vi "_CSM - Read Log Filter Rules - v1.0.vi"(5 "Section Name(\"LogFilterRules\")":string="LogFilterRules", 7 "error in (no error)":errorcluster) -> (1 "error out":errorcluster, 3 "Rules-v1":T1)   [LabVIEW 2017, in "INI-Static-Variable-Support.lvlib"]
uses:
  INI-Static-Variable-Support.lvlib
  <userlib>/_NEVSTOP/Communicable State Machine(CSM)/_Support/Typedef/_CSM_GlobalLog Filter Rules - v1.0.ctl
  <userlib>/_NEVSTOP/Communicable State Machine(CSM)/_Support/Typedef/_CSM_GlobalLog_MSG_TYPE.ctl
  <userlib>/_NEVSTOP/Communicable State Machine(CSM)/_Support/Typedef/_CSM_GlobalLog_STATE_TYPE.ctl
  _fgv-oper.ctl
  <userlib>/_NEVSTOP/Communicable State Machine(CSM)/_Support/ChangeFlag/ChangeFlag-Read.vi
  <userlib>/_NEVSTOP/Communicable State Machine(CSM)/_Support/ChangeFlag/ChangeFlagDB.vi
  <userlib>/_NEVSTOP/Communicable State Machine(CSM)/Communicable State Machine.lvlib
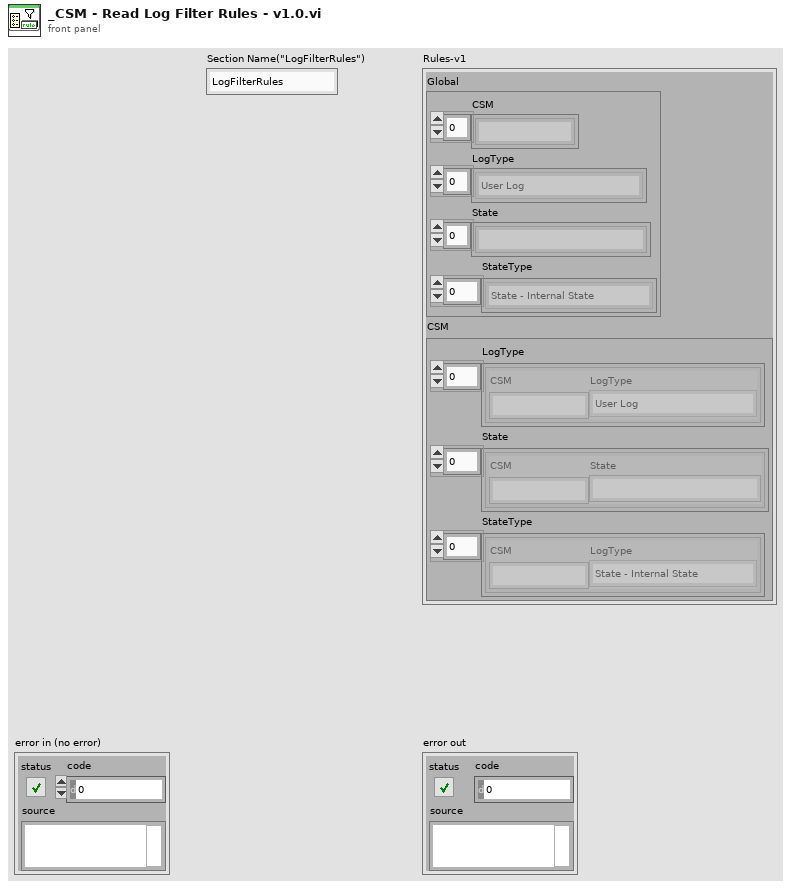
[diagram p1: front panel]
types:
  T1 = typedef "Communicable State Machine.lvlib/_CSM_GlobalLog Filter Rules - v1.0.ctl" = cluster{"Global":cluster{"CSM":string[], "LogType":T2[], "State":string[], "StateType":T3[]}, "CSM":cluster{"LogType":cluster{"CSM":string, "LogType":T2}[], "State":cluster{"CSM":string, "State":string}[], "StateType":cluster{"CSM":string, "LogType":T3}[]}}
  T2 = typedef "Communicable State Machine.lvlib/_CSM_GlobalLog_MSG_TYPE.ctl" = enum16{"User Log", "State Change", "Status", "Interrupt", "Register", "Unregister", "Error Log", "Module Created", "Module Destroyed"}
  T3 = typedef "Communicable State Machine.lvlib/_CSM_GlobalLog_STATE_TYPE.ctl" = enum16{"State - Internal State", "State - External Message", "State - Response", "State - Complete"}
  T4 = typedef "INI-Static-Variable-Support.lvlib/_fgv-oper.ctl" = enum16{"Read", "Write", "Sync", "Sessions", "List Keys", "Load", "List Files", "List Variables", "List Permanent Variables", "Mark Temp Variable as Permenent", "unload", "INIConfig(Memory)", "Reset", "Restore Variable Value"}
  T5 = typedef "LabVIEW-Config.lvlib/Config.ctl" = cluster{"Path":path, "Lines":string[], "Tokens":T6[], "Modified?":bool}
  T6 = typedef "LabVIEW-Config.lvlib/LineToken.ctl" = enum8{"comment", "section", "key", "more"}
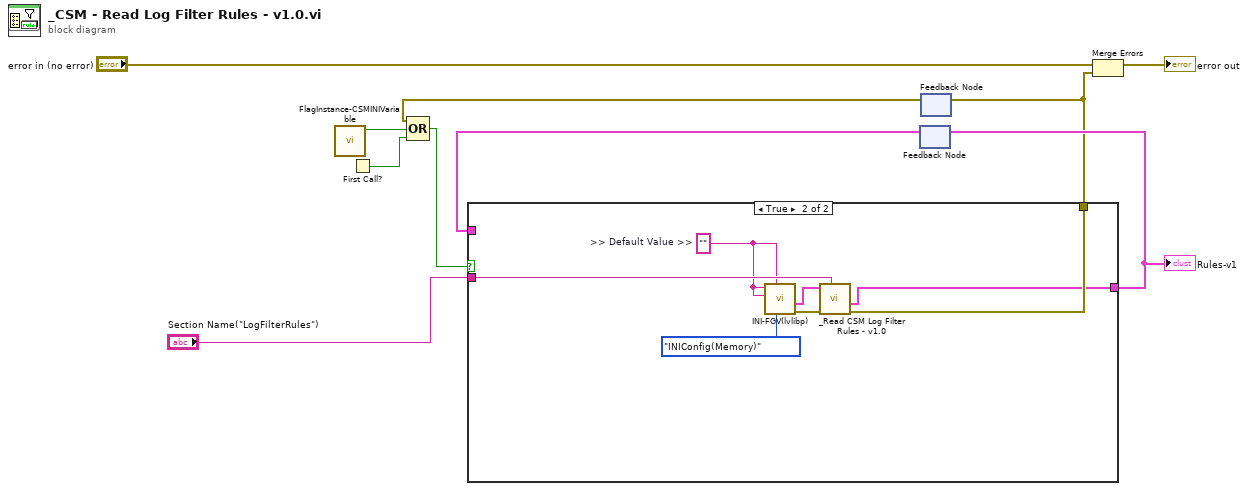
[diagram p0: block diagram]
diagram:
  n1 = call "FlagInstance-CSMINIVariable.vi"() -> ("Changed"=w1:bool)  [unwired: 10 in, 1 out]
  n2 = First Call?() -> (First Call?: T/F=w2:bool)
  n3 = feedback #1() -> (w7:T1)  [unwired: 1 in]
  n4 = feedback #2() -> (w5:errorcluster)  [unwired: 1 in]
  n5 = Compound Arithmetic op=OR(w5, w1, w2) -> (w4:bool)
  n6 = case shown="True" w4 {
    tunnel: [_ w16] -> w6
    tunnel: [w11 w15] -> w8
    tunnel: w7 -> [w11 _]
    tunnel: "Section Name(\"LogFilterRules\")" -> [_ w13]
    frame False {
    }
    frame True {
      w12 = ""  # >> Default Value >>
      n7 = call "INI-FGV(lvlibp).vi"("Enum"=_fgv-oper."INIConfig(Memory)", "Prefered Section"=w12, ">> Default Value >>"=w12, ">> Variable Name >>"=w12) -> ("error out"=w17:errorcluster, "INIConfig"=w14:T5)  [unwired: 4 in, 2 out]
      n8 = call "_Read CSM Log Filter Rules - v1.0.vi"("Section Name"=w13, "error in (no error)"=w17, "Config"=w14) -> ("error out"=w16:errorcluster, "Rules-v1"=w15:T1)  [unwired: 5 in, 2 out]
    }
  }
  "Rules-v1" <- w8
  n9 = feedback-in #1(w8) -> ()
  n10 = feedback-in #2(w6) -> ()
  n11 = Merge Errors("error in (no error)", w6) -> (→"error out":errorcluster)
